vi "FPGA Main.vi"() -> ()   [LabVIEW 2016]
uses:
  Sub VIs for FPGA/SubVIs needed for the customize FPGA VI/Utilities/Start Boolean.ctl
  <vilib>/Platform/TimedLoop/XDataNode/timing_clust.ctl
  <vilib>/Platform/TimedLoop/XDataNode/nitl_modes.ctl
  <vilib>/Platform/TimedLoop/XDataNode/wakeup.ctl
  <vilib>/rvi/Emulation/niFpgaGetClockAttributes.vi
  <vilib>/rvi/Emulation/niFpgaSctlEmulationGetInTimedLoop.vi
  <vilib>/rvi/Emulation/niFpgaEmulationReportErrorSimple.vi
  <vilib>/rvi/eio/common/nirviEmuTemplateMethod_errors.vi
  <vilib>/rvi/Emulation/niFpgaCriticalErrorInLSC.vi
  <vilib>/rvi/Emulation/niFpgaProcessEmulError.vi
  <vilib>/rvi/Emulation/niFpgaEmulationIsFPGAContextNoSignature.vi
  <vilib>/rvi/errors/niFpgaSetErrorForExecOnDevCompSimple.vi
  <vilib>/rvi/eio/common/nirviEmuReportErrorAndStop.vi
  <vilib>/rvi/DataTransferAndStorage/Container/Common/niFpgaContainerGetUniqueNameForEmu.vi
  <vilib>/rvi/FIFO/Fifo_Resource/nirvififoEmulationSetSize.vi
  <vilib>/rvi/FIFO/Fifo_Resource/nirviFifoEmulationQueueMgr.vi
  <instcachedir>/0/nirviFifoEmulationQueueMgr_E5CAEC123FF24DC58D834DCA3CDAA9B5.lvgen/nirviFifoEmulationQueueMgr_E5CAEC123FF24DC58D834DCA3CDAA9B5_000.vi
  <vilib>/Utility/error.llb/Clear Errors.vi
  <vilib>/rvi/FIFO/Fifo_Resource/nirvififoEmulationCreateLock.vi
  <vilib>/rvi/FIFO/Fifo_Resource/nirvififoEmulationObtainLock.vi
  <vilib>/rvi/FIFO/Fifo_Resource/nirvififoEmulationReleaseLock.vi
  <vilib>/rvi/occurrence/nirviWaitOnOccurrenceBase.vi
  <vilib>/rvi/errors/nirviReportUnexpectedCaseInternalError.vi
  <vilib>/rvi/errors/nirviReportUnexpectedCaseInternalError (U32).vi
  <vilib>/rvi/FIFO/Fifo_Resource/nirvififoEmulationDetermineInputValidOut.vi
  <vilib>/rvi/DataTransferAndStorage/Container/Common/niFpgaContainerExecOnDevCompGetState.vi
  <vilib>/rvi/interface/RandomDataEmulation/niFpgaRandomDataHandleErrors.vi
  <vilib>/rvi/DataTransferAndStorage/Container/Common/niFpgaContainerSetEmuInfo.vi
  <instcachedir>/0/nirviFifoEmulationQueueMgr_E5CAEC123FF24DC58D834DCA3CDAA9B5.lvgen/nirviFifoEmulationQueueMgr_E5CAEC123FF24DC58D834DCA3CDAA9B5_001.vi
  <vilib>/rvi/Memory/Memory_Emulation/niFpgaMemoryEmulationCacheClearOnFirstRun.vi
  <vilib>/rvi/Memory/Memory_Emulation/nirvimemoryEmulationManagerCache_MakeExclusive.vi
  <vilib>/rvi/Memory/Memory_Emulation/niFpgaMemoryEmulationValidateCache.vi
  <vilib>/rvi/Memory/Memory_Emulation/nirvimemoryEmulationManagerCache_InsertValue.vi
  <vilib>/rvi/Memory/Memory_Emulation/nirvimemoryEmulationManagerCache_ReleaseExclusive.vi
  <vilib>/rvi/Memory/Memory_Emulation/nirvimemoryEmulationManagerCache_GetValue.vi
  <vilib>/rvi/Memory/Memory_Emulation/nirvimemoryEmulationManagerCache_SetValue.vi
  <vilib>/eio/EIONode/EIONode.xnode
  <vilib>/rvi/DataTransferAndStorage/Container/XNode/niFpgaContainer.xnode
  <vilib>/rvi/FIFO/Fifo_Resource/nirvififoEmulationRead.vi
  <vilib>/rvi/FIFO/Fifo_Resource/nirvififoEmulationWrite.vi
  <vilib>/rvi/FIFO/Fifo_Resource/niFpgaFifoEmulationRefIn.vi
  <vilib>/eio/EIOMethodNode/EIOMethodNode.xnode
  <vilib>/rvi/LocalResourceManager/LocalResourceManager.xnode
  <vilib>/rvi/DataTransferAndStorage/Register/Emulation/niFpgaRegisterEmulationRefIn.vi
  <vilib>/platform/TimedLoop/XDataNode/XDataNode.xnode
  <vilib>/Platform/TimedLoop/XDataNode/XDNodeRunTimeDep.lvlib
panel:
  in  "MotorsON":bool=TRUE
  out "ODrive Encoder ready":bool
  in  "SPI.SPI.DATO":u16
  out "SPI.SPI.DATI":u16
  in  "SPI.SPI.CNFG":u16 format="%016b"
  in  "SPI.SPI.CNT":u16
  in  "SPI.SPI.GO":T1
  out "SPI.SPI.STAT":u8 format="%08b"
  in  "DIO.SPI_CS3:0.OUT":u8 format="%08b"
  in  "DIO.SPI_CS3:0.DIR":u8 format="%08b"
  out "DIO.SPI_CS3:0.IN":u8 format="%08b"
  in  "IRQ.TIMER.SETTIME":T1
  in  "IRQ.TIMER.WRITE":u32
  out "IRQ.TIMER.READ":u32
  out "SYS.AI.RDY":bool
  out "SYS.ACC.RDY":bool
  out "SYS.RDY":bool
  in  "ODrive RT Control":bool
  out "Position Axis1":i16
  out "Velocity Axis0":i16
  out "ODrive State":u8
  out "ODrive Error Flags":bool[](array[boolean])
  out "ODrive Errors":u32
  out "IMU_String":u8[](array[numeric])
  out "User Button":bool
  in  "Comm LED Red":bool
  in  "Comm LED Green":bool
  in  "IMU ON?":bool
  # "SPI"
  # "System"
  # "FPGA Timer"
  # "SPI CS DIO"
  # "RC"
  # "LEDS and user button"
  # "IMU"
  # "UWB"
  # "LQR"
  # "Steering"
  # "Rear wheel"
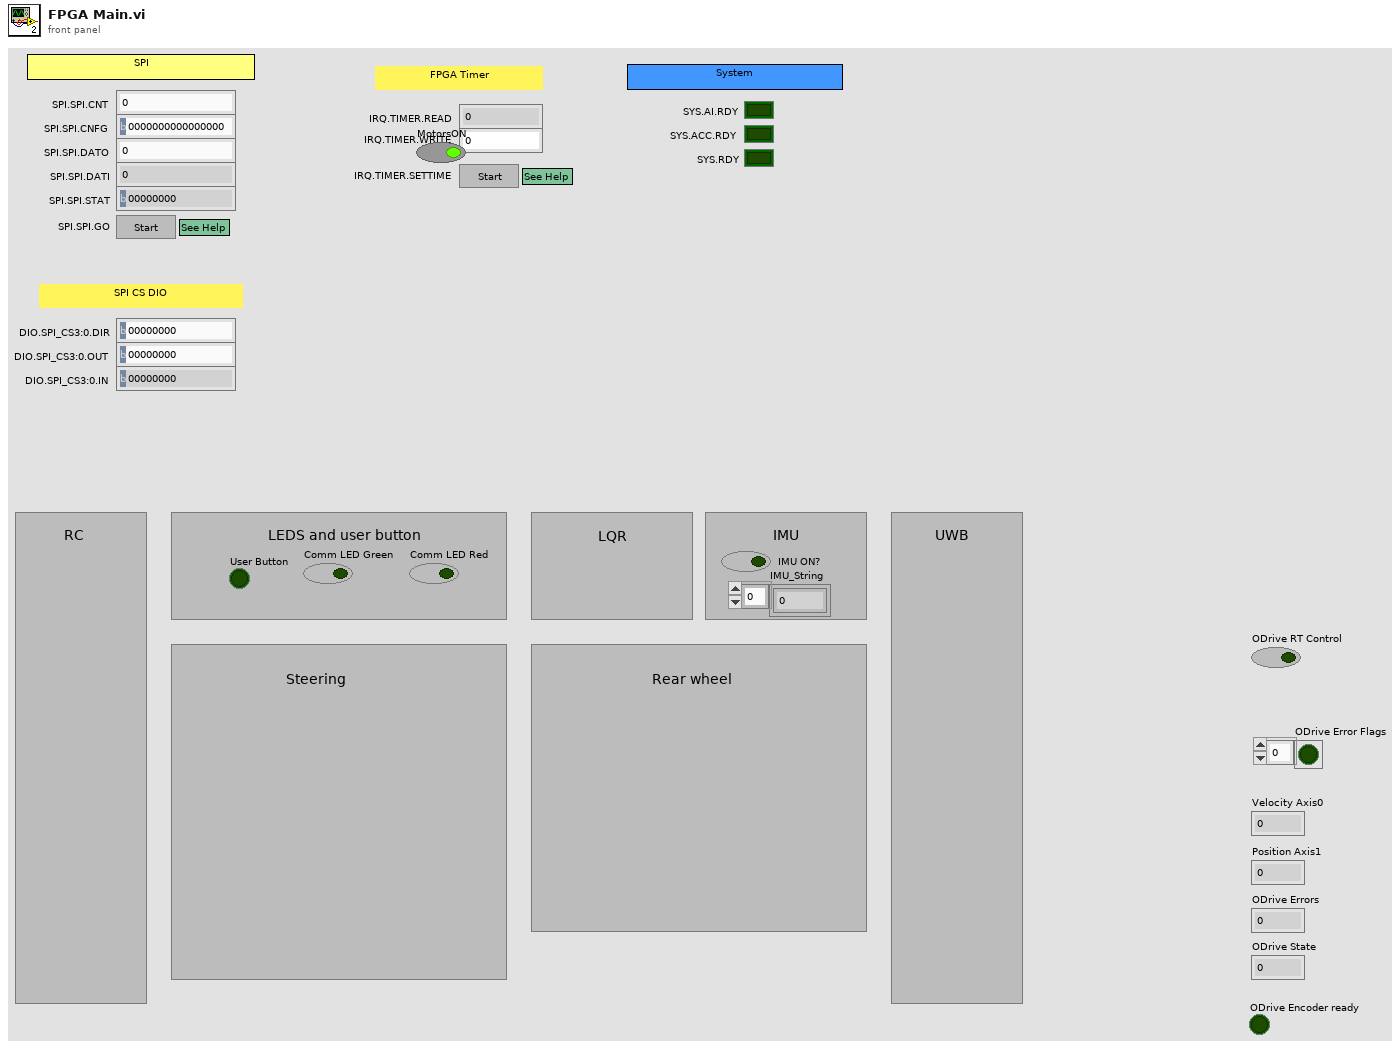
[diagram p1: front panel]
types:
  T1 = typedef "Start Boolean.ctl" = bool
  T2 = cluster{"ASCII command":u8, "Flags":u8, "Value":i16}
  T3 = typedef "XDNodeRunTimeDep.lvlib/timing_clust.ctl" = cluster{"Expected End [f-1]":u64, "Actual End [f-1]":u64, "Finished Late? [f-1]":bool, "Expected End [i-1]":u64, "Actual End [i-1]":u64, "Finished Late? [i-1]":bool, "Expected Start [i]":u64, "Actual Start [i]":u64, "Expected Start [f]":u64, "Actual Start [f]":u64, "Source Name":string, "Structure Name":string, "Period":i64, "Deadline":i64, "Offset":i64, "Start":i64, "Priority":i32, "Timeout":i32, "Mode":T4, "Wakeup Reason":T5, "Error":errorcluster, "Source Type":string, "Secondary Source Type":string, "Global End Time":u64, "Global Start Time":u64, "Frame Duration":u64, "Iteration Duration":u64, "Assigned CPU":i32, "I/O Scan Engine Mode":u32}
  T4 = typedef "XDNodeRunTimeDep.lvlib/nitl_modes.ctl" = enum32{"No Change", "Process missed periods, maintain original phase", "Discard missed periods, maintain original phase", "Process missed periods, ignore original phase", "Discard missed periods, ignore original phase"}
  T5 = typedef "XDNodeRunTimeDep.lvlib/wakeup.ctl" = enum32{"Normal", "Aborted", "Asynchronous wakeup", "Timing source error", "Timed loop error", "Timeout"}
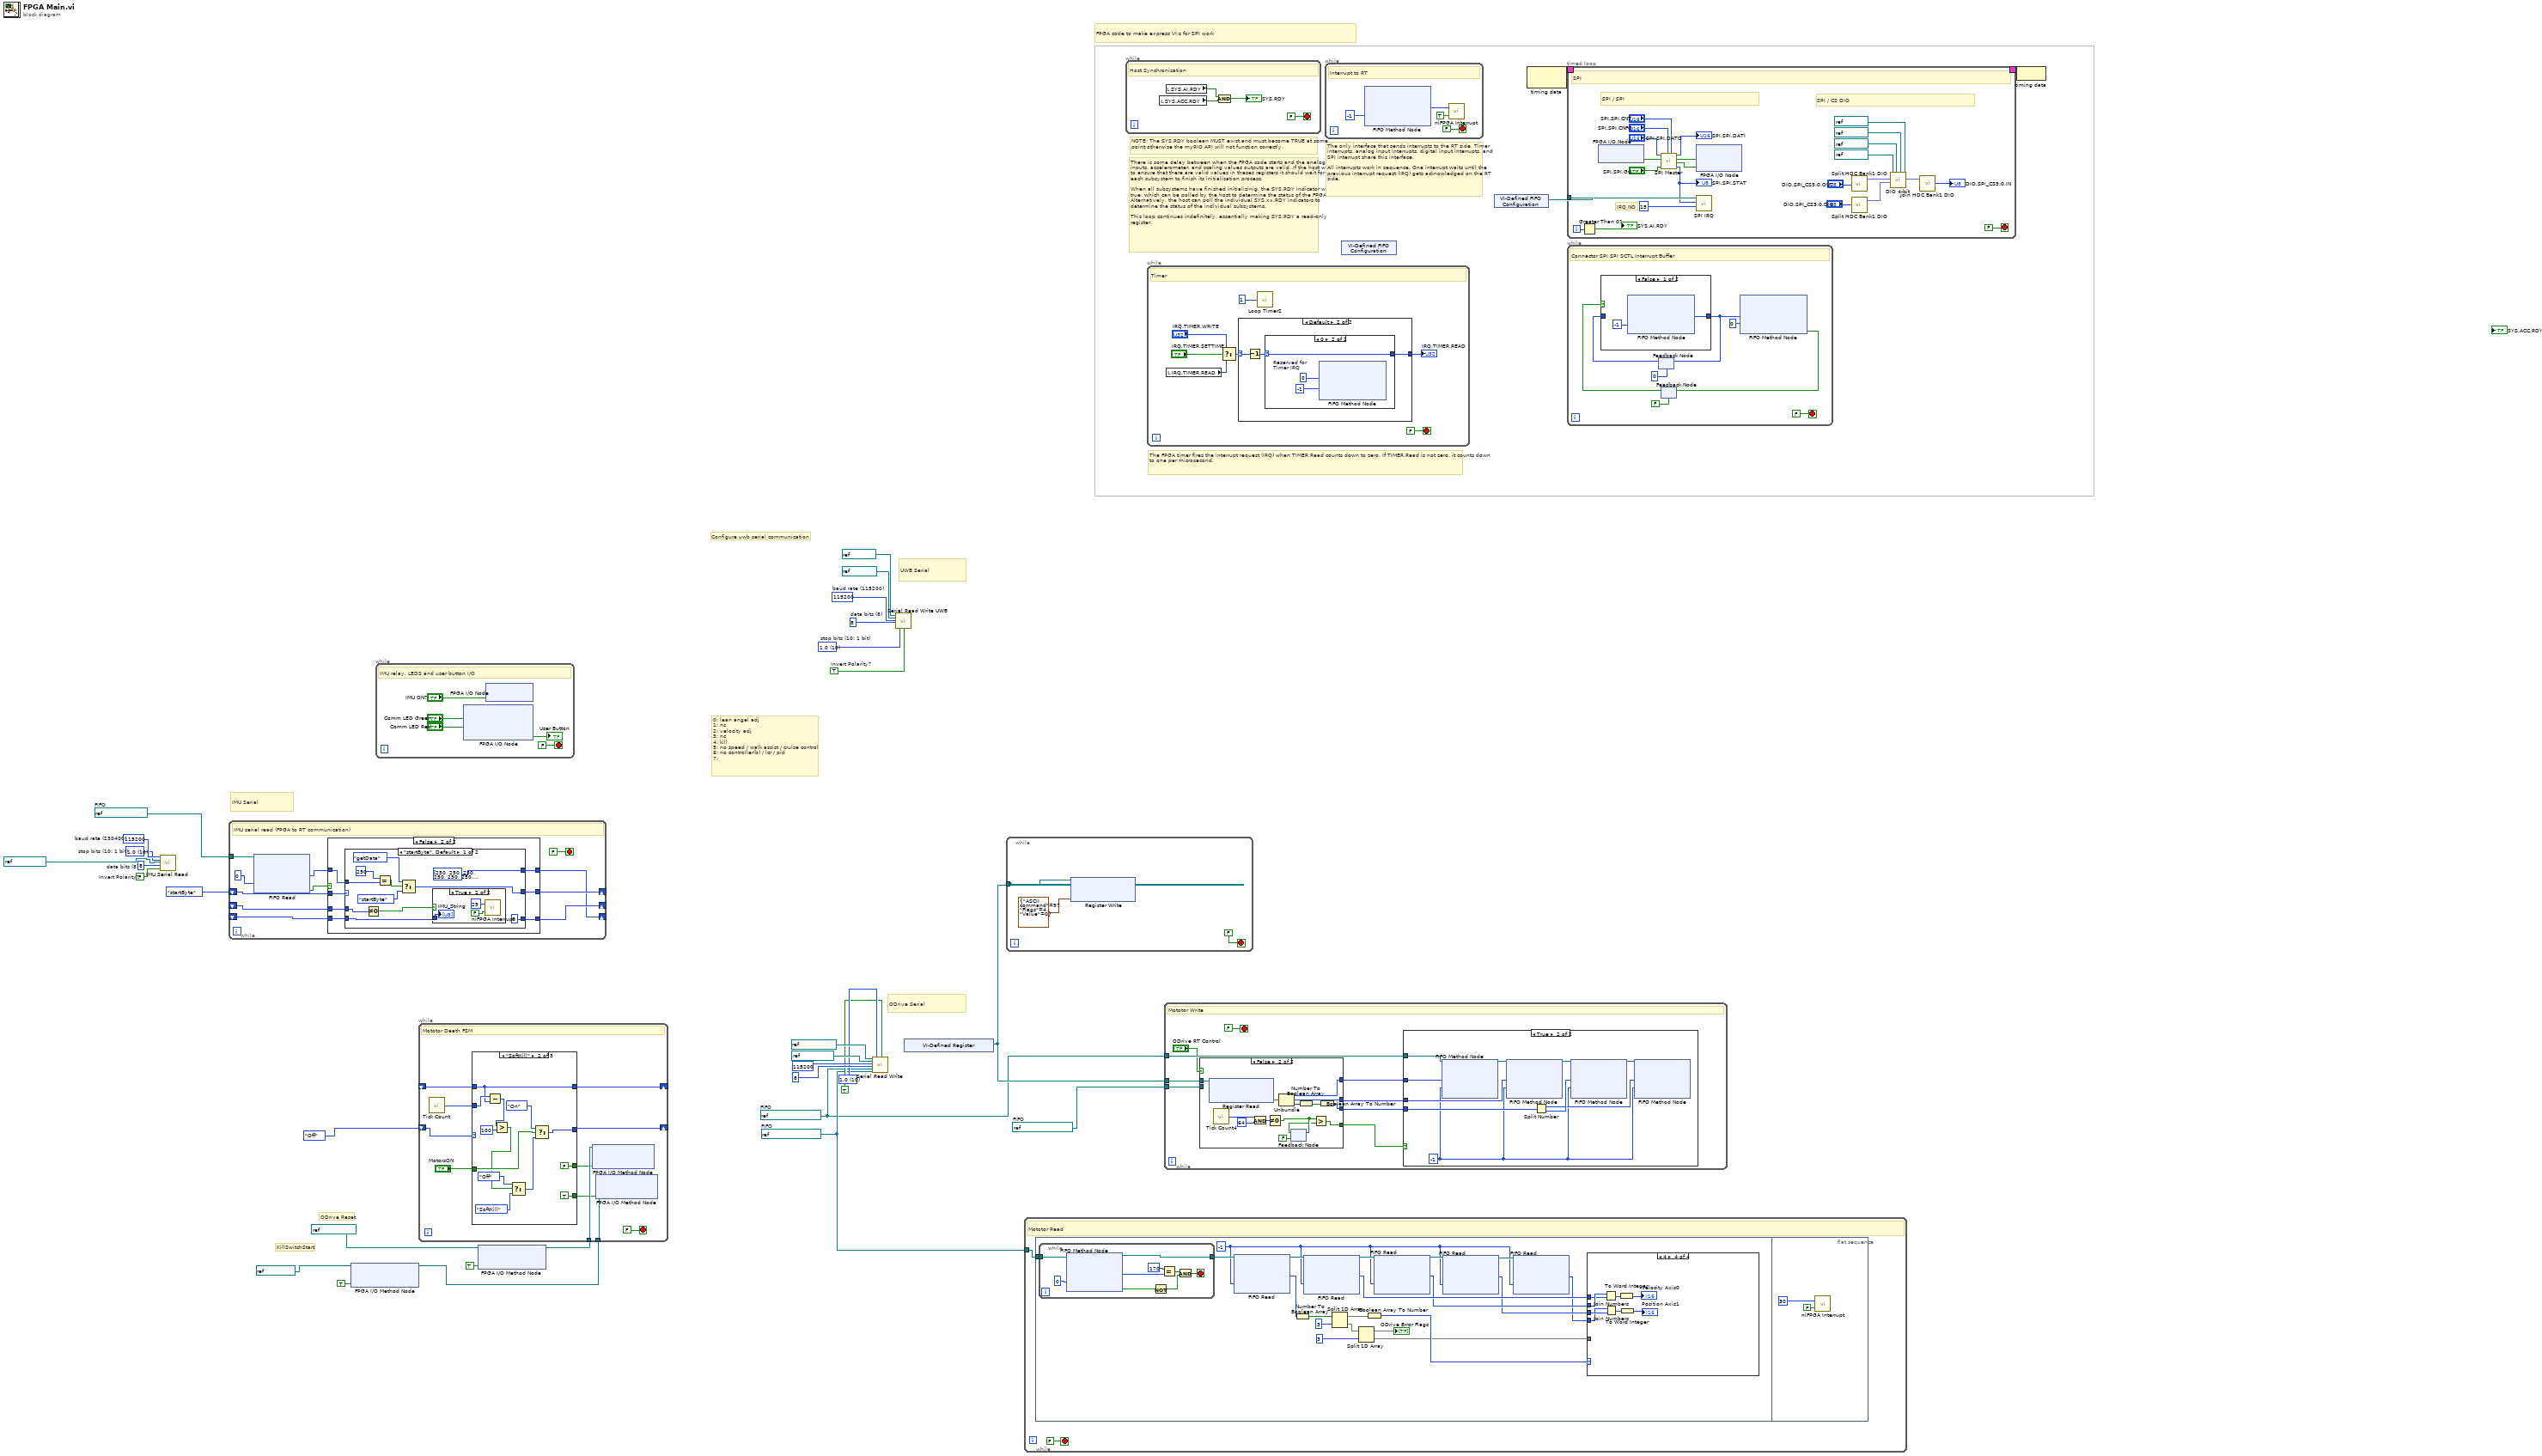
[diagram p0: block diagram]
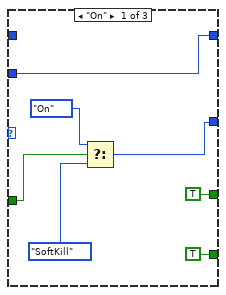
[diagram p2: hidden frame]
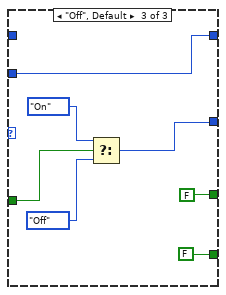
[diagram p3: hidden frame]
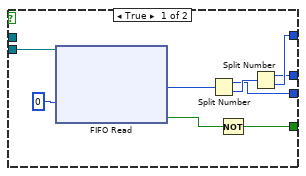
[diagram p8: hidden frame]
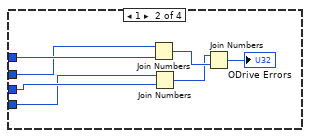
[diagram p10: hidden frame]
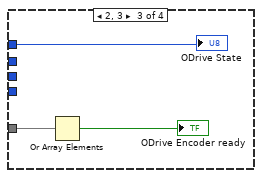
[diagram p11: hidden frame]
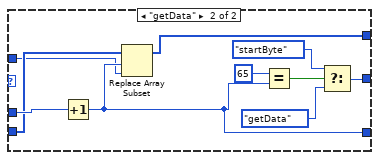
[diagram p14: hidden frame]
diagram:
  w18 = refnum<k21> "RT to ODrive FIFO"  # FIFO
  w23 = u16 10 items=["1.0"=10, "1.5"=15, "2.0"=20] ("stop bits (10: 1 bit)")
  w21 = refnum<k21> "Read FIFO ODrive"  # FIFO
  w19 = refnum<k21> "Write FIFO ODrive"  # FIFO
  w32 = refnum<k21> "Read FIFO IMU"  # FIFO
  w28 = FALSE  # Invert Polarity?
  w29 = 8  # data bits (8)
  w30 = u16 10 items=["1.0"=10, "1.5"=15, "2.0"=20]  # stop bits (10: 1 bit)
  w31 = u32 115200  # baud rate (230400)
  w1 = TRUE  # Invert Polarity?
  w2 = u16 10 items=["1.0"=10, "1.5"=15, "2.0"=20]  # stop bits (10: 1 bit)
  w3 = 8  # data bits (8)
  w4 = u32 115200  # baud rate (115200)
  # "KillSwitchStart"
  # "ODrive Reset"
  # "FPGA code to make express VI:s for SPI work"
  # "The FPGA timer fires the interrupt request (IRQ) when TIMER.Read counts down to zero. If TIMER.Read is not zero, it counts down to one per microsecond."
  # "The only interface that sends interrupts to the RT side. Timer interrupts, analog input interrupts, digital input interrupts, and SPI interrupt share this interface.\n\nAll interrupts work in sequence. One interrupt waits until the previous interrupt request (IRQ) gets acknowledged on the RT side."
  # "NOTE: The SYS.RDY boolean MUST exist and must become TRUE at some point otherwise the myRIO API will not function correctly."
  # "There is some delay between when the FPGA code starts and the analog inputs, accelerometer, and scaling values outputs are valid. If the host wants to ensure that there are valid values in theses registers it should wait for each subsystem to finish its initialization process. \n\nWhen all subsystems have finished initializinig, the SYS.RDY indicator will be true, which can be polled by the host to determine the status of the FPGA. Alternatively, the host can poll the individual SYS.xx.RDY indicators to determine the status of the individual subsystems.\n\nThis loop continues indefinitely, essentially making SYS.RDY a read-only register."
  # "0: lean angel adj\n1: nc\n2: velocity adj\n3: nc\n4: kill\n5: no speed / walk assist / cruise control\n6: no controller(b) / lcr / pid\n7:"
  # "ODrive Serial"
  # "Configure uwb serial communication"
  # "IMU Serial"
  # "UWB Serial"
  n1 = call "IMU Serial Read.vi"("baud rate (230400)"=w31, "stop bits (10: 1 bit)"=w30, "Receive"=refnum<k21> "MXP/DIO5", "data bits (8)"=w29, "Invert Polarity?"=w28) -> ()  [unwired: 11 in]
  n2 = while {
    shift-right: [w42] -> _
    shift-left: enum16{"startByte", "getData"}."startByte" -> [w43]
    shift-right: [w38] -> _
    shift-left: _ -> [w39]
    shift-right: [w41] -> _
    shift-left: _ -> [w40]
    tunnel: w32 -> [w37]
    stop <- FALSE stop-if-true
    # "IMU serial read (FPGA to RT communication)"
    n3 = xnode ("FIFO Read")("Timeout"=0, "FIFO In"=w37) -> ("Element"=w35:u8, "Timed Out?"=w34:bool)  [unwired: 1 out]
    n4 = case shown="False" w34 {
      tunnel: w43 -> [w46 w54]
      tunnel: [w46 w53] -> w42
      tunnel: [w45 w52] -> w41
      tunnel: w40 -> [w45 w51]
      tunnel: w39 -> [w47 w50]
      tunnel: [w47 w49] -> w38
      tunnel: w35 -> [_ w48]
      frame True {
      }
      frame False {
        n5 = case shown="\"startByte\", Default" w54 {
          tunnel: w48 -> [w65 w70]
          tunnel: [w61 w77] -> w53
          tunnel: [u8[] [250, 250, 250, 250, 250, 250, 250, 250, 250, 250, 250, 250, 250, 250, 250, 250, 250, 250, 250, 250, 250, 250, 250, 250, 250, 250, 250, 250, 250, 250, 250, 250, 250, 250, 250, 250, 250, 250, 250, 250, 250, 250, 250, 250, 250, 0, 0, 0, 0, 0, 0, 0, 0, 0, 0, 0, 0, 0, 0, 0, 0, 0, 0, 0, 0, 0] ("IMU_String") w69] -> w49
          tunnel: [u8 0 w71] -> w52
          tunnel: w51 -> [w58 w78]
          tunnel: w50 -> [w56 w72]
          frame "startByte", Default {
            n6 = Not Equal To 0?(x=w58) -> (x != 0?=w55:bool)
            n7 = Equal?(x=u8 250, y=w65) -> (x = y?=w57:bool)
            n8 = Select(t=enum16{"startByte", "getData"}."getData", s=w57, f=enum16{"startByte", "getData"}."startByte") -> (s? t:f=w61:enum16{"startByte", "getData"})
            n9 = case shown="True" w55 {
              tunnel: w56 -> [_ w68]
              frame False {
              }
              frame True {
                n10 = call <vilib>:"niFPGA Interrupt.vi"("Wait Until Cleared (F)"=FALSE, "IRQ Number (0)"=u8 29) -> ()  [unwired: 1 in]
                "IMU_String" <- w68
              }
            }
          }
          frame "getData" {
            n11 = Increment(x=w78) -> (x+1=w71:u8)
            n12 = Replace Array Subset(array=w72, new element=w70, index=w71) -> (w69:u8[])
            n13 = Equal?(x=u8 65, y=w71) -> (x = y?=w75:bool)
            n14 = Select(t=enum16{"startByte", "getData"}."startByte", s=w75, f=enum16{"startByte", "getData"}."getData") -> (s? t:f=w77:enum16{"startByte", "getData"})
          }
        }
      }
    }
  }
  n15 = xnode "FPGA I/O Method Node"("FPGA I/O In"=refnum<k21> "DIO/DIO0" ("Transmit"), "Enable"=TRUE) -> ("FPGA I/O Out"=w7:refnum<k21>)
  n16 = while {
    stop <- FALSE stop-if-true
    # "IMU relay, LEDS and user button I/O"
    n17 = xnode "FPGA I/O Node"("Comm LED Green"="Comm LED Green", "Comm LED Red"="Comm LED Red") -> ("User Button"=→"User Button":bool)  [unwired: 3 in, 3 out]
    n18 = xnode "FPGA I/O Node"("DIO/DIO3"="IMU ON?") -> ()  [unwired: 1 in, 1 out]
  }
  n19 = xnode "FPGA I/O Method Node"("FPGA I/O In"=refnum<k21> "MXP/DIO15" ("Transmit"), "Enable"=TRUE) -> ("FPGA I/O Out"=w10:refnum<k21>)
  n20 = while {
    shift-right: [w84] -> _
    shift-left: enum16{"On", "SoftKill", "Off"}."Off" -> [w93]
    shift-right: [w92] -> _
    shift-left: _ -> [w90]
    tunnel: w10 -> [w89]
    tunnel: w7 -> [w88]
    stop <- FALSE stop-if-true
    # "Mototor Death FSM"
    n21 = call "Tick Count"() -> ("Tick Count(mSec)"=w91:u16)
    n22 = case shown="\"SoftKill\"" w93 {
      tunnel: [w101 w102 w121] -> w92
      tunnel: w91 -> [w101 w103 w121]
      tunnel: w90 -> [_ w102 _]
      tunnel: [TRUE FALSE FALSE] -> w87
      tunnel: [TRUE TRUE FALSE] -> w86
      tunnel: "MotorsON" -> [w98 w112 w118]
      tunnel: [w95 w110 w115] -> w84
      frame "On" {
        n23 = Select(t=enum16{"On", "SoftKill", "Off"}."On", s=w98, f=enum16{"On", "SoftKill", "Off"}."SoftKill") -> (s? t:f=w95:enum16{"On", "SoftKill", "Off"})
      }
      frame "SoftKill" {
        n24 = Subtract(x=w103, y=w102) -> (x-y=w109:u16)
        n25 = Greater?(x=w109, y=u16 100) -> (0:w107:bool)
        n26 = Select(t=enum16{"On", "SoftKill", "Off"}."Off", s=w107, f=enum16{"On", "SoftKill", "Off"}."SoftKill") -> (s? t:f=w104:enum16{"On", "SoftKill", "Off"})
        n27 = Select(t=enum16{"On", "SoftKill", "Off"}."On", s=w112, f=w104) -> (s? t:f=w110:enum16{"On", "SoftKill", "Off"})
      }
      frame "Off", Default {
        n28 = Select(t=enum16{"On", "SoftKill", "Off"}."On", s=w118, f=enum16{"On", "SoftKill", "Off"}."Off") -> (s? t:f=w115:enum16{"On", "SoftKill", "Off"})
      }
    }
    n29 = xnode "FPGA I/O Method Node"("FPGA I/O In"=w89, "Data"=w87) -> ()  [unwired: 1 out]
    n30 = xnode "FPGA I/O Method Node"("FPGA I/O In"=w88, "Data"=w86) -> ()  [unwired: 1 out]
  }
  n31 = call "Serial Read Write.vi"("Transmit"=refnum<k21> "MXP/DIO10", "Receive"=refnum<k21> "MXP/DIO8", "baud rate (115200)"=u32 115200, "data bits (8)"=8, "Transmit FIFO In"=w19, "Receive FIFO In"=w21, "stop bits (10: 1 bit)"=w23, "Invert Polarity?"=TRUE) -> ()  [unwired: 12 in]
  n32 = call "Serial Read Write UWB.vi"("Transmit"=refnum<k21> "I2C SCL", "Receive"=refnum<k21> "I2C SDA", "baud rate (115200)"=w4, "data bits (8)"=w3, "stop bits (10: 1 bit)"=w2, "Invert Polarity?"=w1) -> ()  [unwired: 14 in]
  n33 = xnode "VI-Defined Register"() -> ("Register Out"=w20:refnum<k21>)
  n34 = while {
    tunnel: [w123] -> _
    tunnel: w20 -> [w123]
    stop <- FALSE stop-if-true
    n35 = xnode ("Register Write")("Data"=T2 {"ASCII command"=97, "Flags"=4, "Value"=0}, "Register In"=w123) -> ()  [unwired: 1 out]
  }
  n36 = while {
    tunnel: w21 -> [w126]
    stop <- FALSE stop-if-true
    # "Mototor Read"
    n37 = flat-sequence {
      tunnel: w126 -> [w133]
      frame #0 {
        w131 = -1 ("Timeout")
        n38 = while {
          tunnel: w133 -> [w166]
          tunnel: [w165] -> w132
          stop <- w167 stop-if-true
          n39 = xnode ("FIFO Method Node")("Timeout"=0, "FIFO In"=w166) -> ("Element"=w171:u8, "Timed Out?"=w172:bool, "FIFO Out"=w165:refnum<k21>)
          n40 = Not(x=w172) -> (.not. x?=w169:bool)
          n41 = Equal?(x=u8 170, y=w171) -> (x = y?=w168:bool)
          n42 = And(x=w168, y=w169) -> (x .and. y?=w167:bool)
        }
        n43 = xnode ("FIFO Read")("Timeout"=w131, "FIFO In"=w132) -> ("Element"=w142:u8, "FIFO Out"=w146:refnum<k21>)  [unwired: 1 out]
        n44 = Number To Boolean Array(number=w142) -> (Boolean array=w138:bool[])
        n45 = xnode ("FIFO Read")("Timeout"=w131, "FIFO In"=w146) -> ("Element"=w137:u8, "FIFO Out"=w145:refnum<k21>)  [unwired: 1 out]
        n46 = Split 1D Array(array=w138, index=3) -> (first subarray=w140:bool[], second subarray=w130:bool[])
        n47 = Split 1D Array(array=w130, index=3) -> (first subarray=→"ODrive Error Flags":bool[], second subarray=w127:bool[])
        n48 = Boolean Array To Number(Boolean array=w140) -> (number=w139:u8)
        n49 = xnode ("FIFO Read")("Timeout"=w131, "FIFO In"=w145) -> ("Element"=w136:u8, "FIFO Out"=w144:refnum<k21>)  [unwired: 1 out]
        n50 = xnode ("FIFO Read")("Timeout"=w131, "FIFO In"=w144) -> ("Element"=w135:u8, "FIFO Out"=w143:refnum<k21>)  [unwired: 1 out]
        n51 = xnode ("FIFO Read")("Timeout"=w131, "FIFO In"=w143) -> ("Element"=w134:u8)  [unwired: 2 out]
        n52 = case shown="4" w139 {
          tunnel: w137 -> [_ w153 w156 w163]
          tunnel: w136 -> [_ w152 _ w164]
          tunnel: w135 -> [_ w151 _ w162]
          tunnel: w134 -> [_ w150 _ w161]
          tunnel: w127 -> [_ _ w155 _]
          frame 0, Default {
          }
          frame 1 {
            n53 = Join Numbers(hi=w152, lo=w153) -> ((hi.lo)=w149:u16)
            n54 = Join Numbers(hi=w150, lo=w151) -> ((hi.lo)=w148:u16)
            n55 = Join Numbers(hi=w148, lo=w149) -> ((hi.lo)=→"ODrive Errors":u32)
          }
          frame 2, 3 {
            n56 = Or Array Elements(Boolean array=w155) -> (logical OR=→"ODrive Encoder ready":bool)
            "ODrive State" <- w156
          }
          frame 4 {
            n57 = Join Numbers(hi=w164, lo=w163) -> ((hi.lo)=w160:u16)
            n58 = Join Numbers(hi=w161, lo=w162) -> ((hi.lo)=w159:u16)
            n59 = To Word Integer(number=w160) -> (16bit integer=→"Velocity Axis0":i16)
            n60 = To Word Integer(number=w159) -> (16bit integer=→"Position Axis1":i16)
          }
        }
      }
      frame #1 {
        n61 = call <vilib>:"niFPGA Interrupt.vi"("Wait Until Cleared (F)"=FALSE, "IRQ Number (0)"=u8 30 ("Element")) -> ()  [unwired: 1 in]
      }
    }
  }
  n62 = while {
    stop <- FALSE stop-if-true
    # "Host Synchronization"
    n63 = local read "SYS.ACC.RDY"() -> (w177:bool)
    n64 = local read "SYS.AI.RDY"() -> (w179:bool)
    n65 = Compound Arithmetic op=AND(w179, w177) -> (→"SYS.RDY":bool)
  }
  n66 = while {
    stop <- FALSE stop-if-true
    # "Timer"
    n67 = local read "IRQ.TIMER.READ"() -> (w183:u32)
    n68 = Select(t="IRQ.TIMER.WRITE", s="IRQ.TIMER.SETTIME", f=w183) -> (s? t:f=w181:u32)
    n69 = case shown="Default" w181 {
      selector: w181 -> [w187 w190]
      tunnel: [w187 w188] -> w180
      frame 0 {
      }
      frame Default {
        n70 = Decrement(x=w190) -> (x-1=w189:u32)
        n71 = case shown="0" w189 {
          selector: w189 -> [w191 w194]
          tunnel: [w191 w194] -> w188
          frame Default {
          }
          frame 0 {
            w193 = u8 0  # Reserved for Timer IRQ
            n72 = xnode ("FIFO Method Node")("Element"=w193, "Timeout"=-1) -> ()  [unwired: 1 in, 2 out]
          }
        }
      }
    }
    "IRQ.TIMER.READ" <- w180
    n73 = call "Loop Timer2"("Count(uSec)"=u8 1 ("Count(mSec)")) -> ()  [unwired: 1 out]
  }
  n74 = while {
    tunnel: w20 -> [w201]
    tunnel: w19 -> [w203]
    tunnel: w18 -> [w199]
    stop <- FALSE stop-if-true
    # "Mototor Write"
    n75 = case shown="False" "ODrive RT Control" {
      tunnel: w201 -> [_ w236]
      tunnel: w199 -> [w221 _]
      tunnel: [w216 w231] -> w196
      tunnel: [w218 w234] -> w198
      tunnel: [w217 w233] -> w197
      tunnel: [w214 w226] -> w195
      frame True {
        n76 = xnode ("FIFO Read")("Timeout"=0, "FIFO In"=w221) -> ("Element"=w220:u32, "Timed Out?"=w215:bool)  [unwired: 1 out]
        n77 = Split Number(x=w220) -> (hi(x)=w216:u16, lo(x)=w219:u16)
        n78 = Not(x=w215) -> (.not. x?=w214:bool)
        n79 = Split Number(x=w219) -> (hi(x)=w217:u8, lo(x)=w218:u8)
      }
      frame False {
        n80 = xnode ("Register Read")("Register In"=w236) -> ("Data"=w235:T2)  [unwired: 1 out]
        n81 = call "Tick Count4"() -> ("Tick Count(mSec)"=w229:u16)
        n82 = And(x=w229, y=u16 64) -> (x .and. y?=w227:u16)
        n83 = Not Equal To 0?(x=w227) -> (x != 0?=w225:bool)
        n84 = Unbundle(w235) -> ("ASCII command"=w234:u8, "Flags"=w233:u8, "Value"=w232:i16)
        n85 = feedback-in #1(w225) -> ()
        n86 = feedback #1(FALSE) -> (w224:bool)
        n87 = Number To Boolean Array(number=w232) -> (Boolean array=w230:bool[])
        n88 = Greater?(x=w225, y=w224) -> (0:w226:bool)
        n89 = Boolean Array To Number(Boolean array=w230) -> (number=w231:u16)
      }
    }
    n90 = case shown="True" w195 {
      tunnel: w203 -> [_ w213]
      tunnel: w198 -> [_ w207]
      tunnel: w197 -> [_ w206]
      tunnel: w196 -> [_ w205]
      frame False {
      }
      frame True {
        w204 = -1 ("Timeout")
        n91 = xnode ("FIFO Method Node")("Element"=w207, "Timeout"=w204, "FIFO In"=w213) -> ("FIFO Out"=w212:refnum<k21>)  [unwired: 1 out]
        n92 = xnode ("FIFO Method Node")("Element"=w206, "Timeout"=w204, "FIFO In"=w212) -> ("FIFO Out"=w211:refnum<k21>)  [unwired: 1 out]
        n93 = Split Number(x=w205) -> (hi(x)=w208:u8, lo(x)=w209:u8)
        n94 = xnode ("FIFO Method Node")("Element"=w209, "Timeout"=w204, "FIFO In"=w211) -> ("FIFO Out"=w210:refnum<k21>)  [unwired: 1 out]
        n95 = xnode ("FIFO Method Node")("Element"=w208, "Timeout"=w204, "FIFO In"=w210) -> ()  [unwired: 2 out]
      }
    }
  }
  n96 = while {
    stop <- FALSE stop-if-true
    # "Interrupt to RT"
    n97 = xnode ("FIFO Method Node")("Timeout"=-1) -> ("Element"=w239:u8)  [unwired: 1 in, 2 out]
    n98 = call <vilib>:"niFPGA Interrupt.vi"("Wait Until Cleared (F)"=TRUE, "IRQ Number (0)"=w239) -> ()  [unwired: 1 in]
  }
  n99 = xnode "VI-Defined FIFO Configuration"() -> ()  [unwired: 1 out]
  n100 = xnode "VI-Defined FIFO Configuration"() -> ("FIFO Out"=w14:refnum<k21>)
  n101 = node-c288() -> (w16:T3)  [unwired: 1 in]
  n102 = timed-loop {
    timing: w16 -> [_]
    timing-out: [_] -> w15
    tunnel: w14 -> [w245]
    i -> [w242]
    stop <- FALSE stop-if-true
    # "IRQ NO"
    # "SPI / CS DIO"
    # "SPI / SPI"
    # "SPI"
    n103 = Greater Than 0?(x=w242) -> (x > 0?=→"SYS.AI.RDY":bool)
    n104 = xnode "FPGA I/O Node"() -> ("SPI MISO"=w262:bool)  [unwired: 1 in, 1 out]
    n105 = call "SPI Master.vi"("Count"="SPI.SPI.CNT", "Configuration"="SPI.SPI.CNFG", "Start?"="SPI.SPI.GO", "MISO"=w262, "Data Out"="SPI.SPI.DATO") -> ("Status"=w243:u8, "SCLK"=w256:bool, "MOSI"=w257:bool, "Data In"=→"SPI.SPI.DATI":u16)  [unwired: 3 in]
    "SPI.SPI.STAT" <- w243
    n106 = xnode "FPGA I/O Node"("SPI MOSI"=w257, "SPI CLK"=w256) -> ()  [unwired: 2 in, 2 out]
    n107 = call "SPI IRQ.vi"("SPI.A.IRQ.NO"=u8 15 ("SPI.SPI.IRQ.NO"), "SPI.STAT"=w243, "FIFO In"=w245) -> ()  [unwired: 9 in]
    n108 = call "Split HDC Bank1 DIO.vi"("IN 7:0"="DIO.SPI_CS3:0.OUT") -> ("OUT 3:0"=w252:fxp<+,4,4>)  [unwired: 2 out]
    n109 = call "Split HDC Bank1 DIO.vi"("IN 7:0"="DIO.SPI_CS3:0.DIR") -> ("OUT 3:0"=w251:fxp<+,4,4>)  [unwired: 2 out]
    n110 = call "DIO 4-bit.vi"("DIO0 Refnum"=refnum<k21> "SPI CS0", "DIO1 Refnum"=refnum<k21> "SPI CS1" ("DIO0 Refnum"), "DIO2 Refnum"=refnum<k21> "SPI CS2" ("DIO0 Refnum"), "DIR 3:0"=w251, "OUT 3:0"=w252, "DIO3 Refnum"=refnum<k21> "SPI CS3" ("DIO0 Refnum")) -> ("IN 3:0"=w250:fxp<+,4,4>)  [unwired: 5 in]
    n111 = call "Join HDC Bank1 DIO.vi"("IN 3:0"=w250) -> ("OUT 7:0"=→"DIO.SPI_CS3:0.IN":u8)  [unwired: 2 in]
  }
  n112 = while {
    stop <- FALSE stop-if-true
    # "Connector SPI SPI SCTL Interrupt Buffer"
    n113 = feedback #2(u8 0 ("Element")) -> (w269:u8)
    n114 = feedback #3(FALSE ("Timed Out?")) -> (w273:bool)
    n115 = case shown="False" w273 {
      tunnel: [w275 w277] -> w270
      tunnel: w269 -> [_ w277]
      frame False {
        n116 = xnode ("FIFO Method Node")("Timeout"=-1) -> ("Element"=w275:u8)  [unwired: 1 in, 2 out]
      }
      frame True {
      }
    }
    n117 = feedback-in #2(w270) -> ()
    n118 = xnode ("FIFO Method Node")("Element"=w270, "Timeout"=0) -> ("Timed Out?"=w271:bool)  [unwired: 1 in, 1 out]
    n119 = feedback-in #3(w271) -> ()
  }
  n120 = node-c288(w15) -> ()
